vi "ApportionFlows.vi"(4 "Press (mBar)":dbl, 5 "Temp (C)":dbl, 7 "C:(%)":dbl, 8 "Q[Total]:(l/min)":dbl) -> (0 "Mdot[Ethane]:(g/min)":dbl, 1 "Q[Ethane]:(l/min)":dbl, 2 "Mdot[N2]:(g/min)":dbl, 3 "Q[N2]:(l/min)":dbl, 6 "Rho[Mix]:Dem(kg/l)":dbl)   [LabVIEW 2016]
uses:
  Anemometry/Anemometry Sub Vis/Controls/GasCombo.ctl
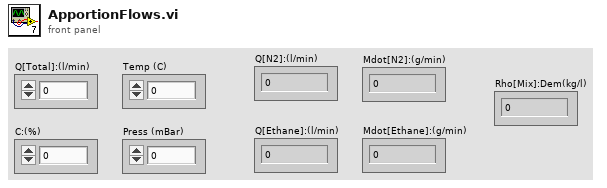
[diagram p1: front panel]
types:
  T1 = typedef "GasCombo.ctl" = string
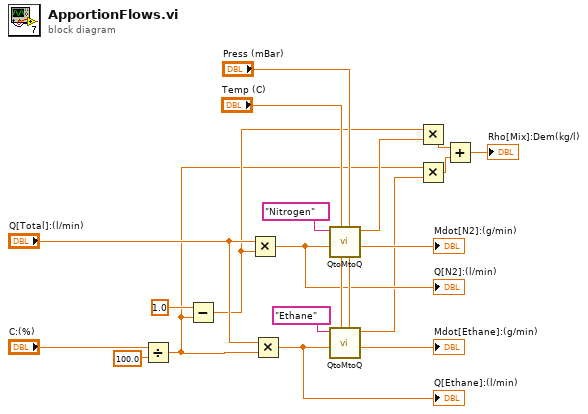
[diagram p0: block diagram]
diagram:
  n1 = Divide(x="C:(%)", y=100.0) -> (x/y=w4:dbl)
  n2 = Subtract(x=1.0, y=w4) -> (x-y=w6:dbl)
  n3 = Multiply(x="Q[Total]:(l/min)", y=w6) -> (x*y=w10:dbl)
  "Q[N2]:(l/min)" <- w10
  n4 = Multiply(x="Q[Total]:(l/min)", y=w4) -> (x*y=w8:dbl)
  "Q[Ethane]:(l/min)" <- w8
  n5 = call "QtoMtoQ.vi"("Pressure"="Press (mBar)", "Temperature"="Temp (C)", "Q in (l/min)"=w10, "Gas"=T1 "Nitrogen") -> ("Mdot out (g/min)"=→"Mdot[N2]:(g/min)":dbl, "Density (kg/m^3) (= g/l)(l/min)"=w7:dbl)  [unwired: 3 in, 1 out]
  n6 = call "QtoMtoQ.vi"("Pressure"="Press (mBar)", "Temperature"="Temp (C)", "Q in (l/min)"=w8, "Gas"=T1 "Ethane") -> ("Mdot out (g/min)"=→"Mdot[Ethane]:(g/min)":dbl, "Density (kg/m^3) (= g/l)(l/min)"=w5:dbl)  [unwired: 3 in, 1 out]
  n7 = Multiply(x=w6, y=w7) -> (x*y=w3:dbl)
  n8 = Multiply(x=w4, y=w5) -> (x*y=w2:dbl)
  n9 = Add(x=w3, y=w2) -> (x+y=→"Rho[Mix]:Dem(kg/l)":dbl)
